vi "Set Drive Motors.vi"(10 "appended array":dbl[](array[numeric]), 11 "Motors In":T1[](array[typedef])) -> (3 "Motors Out":T1[](array[typedef]))   [LabVIEW 2018]
uses:
  <vilib>/Rock Robotics/WPI/MotorControl/WPI_MotorControlDeviceRef.ctl
  <vilib>/Rock Robotics/WPI/MotorControl/WPI_MotorControlType.ctl
  <vilib>/Rock Robotics/SystemInterfaces/DIO/FPGA_DIOPWMChannel.ctl
  <vilib>/Rock Robotics/WPI/PWM/WPI_PWMDeadband.ctl
  <vilib>/Rock Robotics/SystemInterfaces/DIO/FPGA_DIOChannel.ctl
  <vilib>/Rock Robotics/WPI/ThirdParty/Phoenix-LabVIEW/Motor Controller/Controls/CTRE_Phoenix_MotorControl_ControlMode.ctl
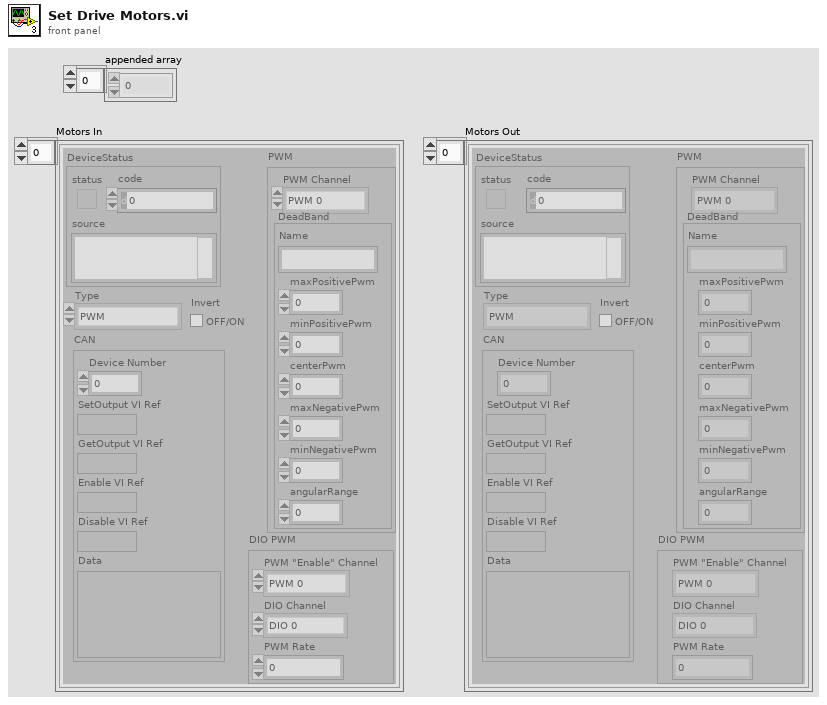
[diagram p1: front panel]
types:
  T1 = typedef "WPI_MotorControlDeviceRef.ctl" = cluster{"DeviceStatus":errorcluster, "Type":T2, "PWM":cluster{"PWM Channel":T3, "DeadBand":T4}, "CAN":cluster{"Device Number":u8, "SetOutput VI Ref":variant, "GetOutput VI Ref":variant, "Enable VI Ref":variant, "Disable VI Ref":variant, "Data":variant}, "Invert":bool, "DIO PWM":cluster{"PWM \"Enable\" Channel":T3, "DIOChannel":T5, "PWM Rate":dbl}}
  T2 = typedef "WPI_MotorControlType.ctl" = enum16{"PWM", "CAN", "DIO PWM"}
  T3 = typedef "FPGA_DIOPWMChannel.ctl" = enum8{"PWM 0", "PWM 1", "PWM 2", "PWM 3", "PWM 4", "PWM 5", "PWM 6", "PWM 7", "PWM 8", "PWM 9", "PWM MXP 0", "PWM MXP 1", "PWM MXP 2", "PWM MXP 3", "PWM MXP 4", "PWM MXP 5", "PWM MXP 6", "PWM MXP 7", "PWM MXP 8", "PWM MXP 9", "Invalid"}
  T4 = typedef "WPI_PWMDeadband.ctl" = cluster{"Name":string, "maxPositivePwm":i32, "minPositivePwm":i32, "centerPwm":i32, "maxNegativePwm":i32, "minNegativePwm":i32, "angularRange":u16}
  T5 = typedef "FPGA_DIOChannel.ctl" = enum8{"DIO 0", "DIO 1", "DIO 2", "DIO 3", "DIO 4", "DIO 5", "DIO 6", "DIO 7", "DIO 8", "DIO 9", "DIO MXP 0", "DIO MXP 1", "DIO MXP 2", "DIO MXP 3", "DIO MXP 4", "DIO MXP 5", "DIO MXP 6", "DIO MXP 7", "DIO MXP 8", "DIO MXP 9", "DIO MXP 10", "DIO MXP 11", "DIO MXP 12", "DIO MXP 13", "DIO MXP 14", "DIO MXP 15", "SPI Port CS1", "SPI Port CS2", "SPI Port CS3", "SPI Port MISO", "SPI Port MOSI", "Invalid"}
  T6 = typedef "CTRE_Phoenix_MotorControl_ControlMode.ctl" = u16
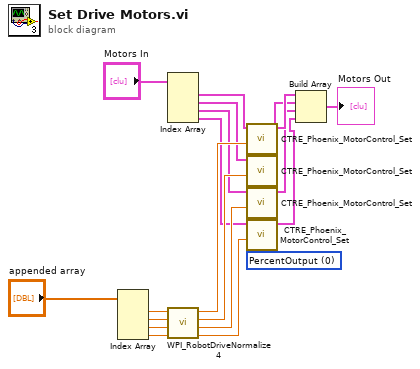
[diagram p0: block diagram]
diagram:
  w16 = T6 0 items=["PercentOutput"=0, "Position"=1, "Velocity"=2, "Current"=3, "Follower"=5, "MotionProfile"=6, "MotionMagic"=7, "MotionProfileArc"=10, "Disabled"=15] ("Control Mode")
  n1 = Index Array(array="appended array") -> (element #1=w14:dbl, element #2=w13:dbl, element #3=w12:dbl, element #4=w11:dbl)  [unwired: 4 in]
  n2 = Index Array(array="Motors In") -> (element #1=w4:T1, element #2=w3:T1, element #3=w2:T1, element #4=w1:T1)  [unwired: 4 in]
  n3 = call <vilib>:"WPI_RobotDriveNormalize 4.vi"("D"=w11, "C"=w12, "B"=w13, "A"=w14) -> ("D'"=w17:dbl, "C'"=w18:dbl, "B'"=w19:dbl, "A'"=w20:dbl)
  n4 = call <vilib>:"CTRE_Phoenix_MotorControl_Set.vi"("Output"=w20, "Control Mode"=w16, "PhoenixMotorControlDevRef"=w4) -> ("PhoenixMotorControlDevRef"=w10:T1)  [unwired: 7 in, 1 out]
  n5 = call <vilib>:"CTRE_Phoenix_MotorControl_Set.vi"("Output"=w19, "Control Mode"=w16, "PhoenixMotorControlDevRef"=w3) -> ("PhoenixMotorControlDevRef"=w9:T1)  [unwired: 7 in, 1 out]
  n6 = call <vilib>:"CTRE_Phoenix_MotorControl_Set.vi"("Output"=w18, "Control Mode"=w16, "PhoenixMotorControlDevRef"=w2) -> ("PhoenixMotorControlDevRef"=w8:T1)  [unwired: 7 in, 1 out]
  n7 = call <vilib>:"CTRE_Phoenix_MotorControl_Set.vi"("Output"=w17, "Control Mode"=w16, "PhoenixMotorControlDevRef"=w1) -> ("PhoenixMotorControlDevRef"=w7:T1)  [unwired: 7 in, 1 out]
  n8 = Build Array(w10, w9, w8, w7) -> (→"Motors Out":T1[])
